vi "pmu_CFG-3 Dulplicate to CFG-2.vi"(8 "error in (no error)":errorcluster, 10 "CFG-3":T5={"PMU ID"=1, "global PMU ID"=1, "time base"=10000000, "nominal frequency"=enum."60 Hz", "reporting rate [fps]"=60, "station name"="", "data format"=15, "phasor channels"=[], "analog channels"=[], "digital channels"=[]} {"data format" format="%016b"; "phasor channels"."phasor unit" items=["Voltage [V]"=0, "Current [A]"=16777216]; "phasor channels"."data modification flag" format="%016b"; "digital channels"."digital unit" format="%08x"}, 11 "CFG-2":T1={"PMU ID"=1, "time base"=10000000, "nominal frequency"=enum."60 Hz", "reporting rate [fps]"=60, "station name"="", "data format"=15, "phasor channels"=[], "analog channels"=[], "digital channels"=[]} {"digital channels"."digital unit" format="%08x"; "analog channels"."analog unit" format="%08x"; "phasor channels"."phasor unit scaling" max=16777215 format="%06x"; "phasor channels"."phasor unit" items=["Voltage [V]"=0, "Current [A]"=16777216]; "data format" format="%016b"}) -> (0 "error out":errorcluster, 3 "CFG-2 output":T1={"PMU ID"=0, "time base"=10000000, "nominal frequency"=enum."60 Hz", "reporting rate [fps]"=60, "station name"="", "data format"=15, "phasor channels"=[], "analog channels"=[], "digital channels"=[]} {"digital channels"."digital unit" format="%08x"; "analog channels"."analog unit" format="%08x"; "phasor channels"."phasor unit scaling" max=16777215 format="%06x"; "phasor channels"."phasor unit" items=["Voltage [V]"=0, "Current [A]"=16777216]; "data format" format="%016b"})   [LabVIEW 2013, in "NI_EP_PMU.lvlib"]
uses:
  <vilib>/addons/Electrical Power/PMU/NI_EP_PMU.lvlib
  <vilib>/addons/Electrical Power/PMU/Common/Controls/pmu_CFG-3 Input.ctl
  <vilib>/addons/Electrical Power/PMU/Common/Controls/pmu_CFG-3 Phasor Channels.ctl
  <vilib>/addons/Electrical Power/PMU/Common/Controls/pmu_CFG-3 Analog Channels.ctl
  <vilib>/addons/Electrical Power/PMU/Common/Controls/pmu_Digital Channel.ctl
  <vilib>/addons/Electrical Power/PMU/Common/Controls/pmu_CFG Input.ctl
  <vilib>/addons/Electrical Power/PMU/Common/Controls/pmu_Phasor Channel.ctl
  <vilib>/addons/Electrical Power/PMU/Common/Controls/pmu_Analog Channel.ctl
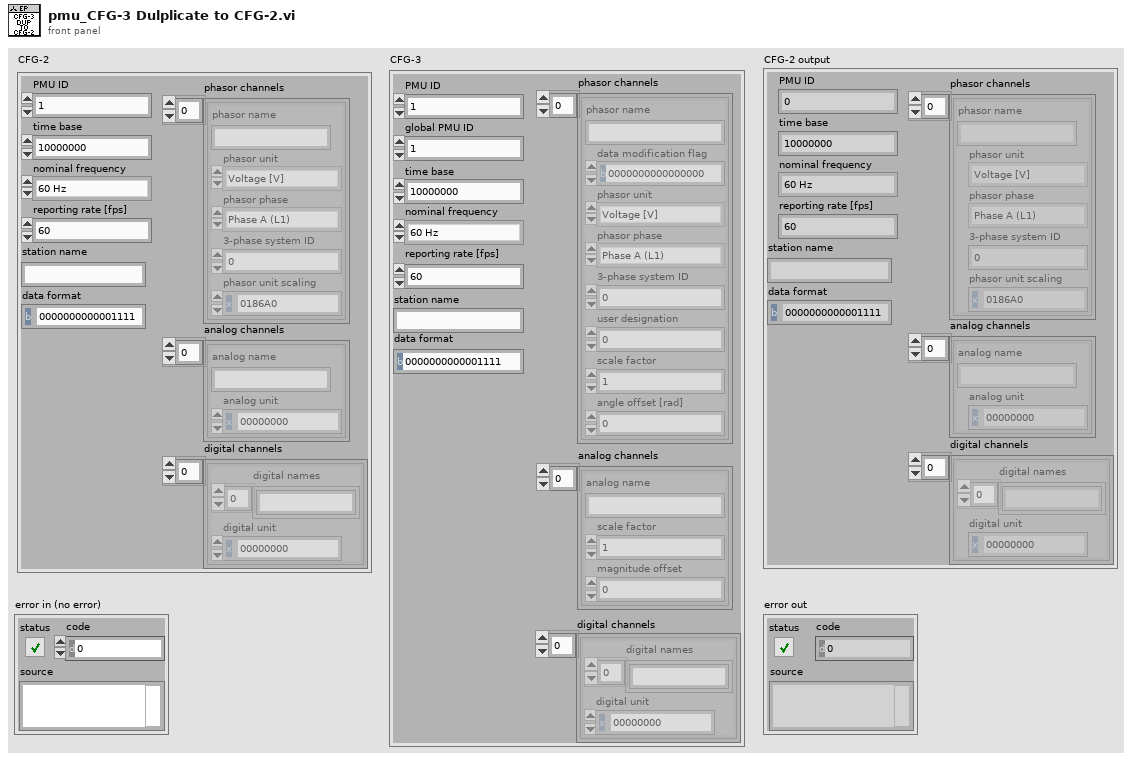
[diagram p1: front panel]
types:
  T1 = typedef "NI_EP_PMU.lvlib/pmu_CFG Input.ctl" = cluster{"PMU ID":u16, "time base":u32, "nominal frequency":enum16{"50 Hz", "60 Hz"}, "reporting rate [fps]":i16, "station name":string, "data format":u16, "phasor channels":T2[], "analog channels":T3[], "digital channels":T4[]}
  T2 = typedef "NI_EP_PMU.lvlib/pmu_Phasor Channel.ctl" = cluster{"phasor name":string, "phasor unit":u32, "phasor phase":enum16{"Phase A (L1)", "Phase B (L2)", "Phase C (L3)", "Phase N", "Positive sequence", "Negative sequence", "Zero sequence"}, "3-phase system ID":u8, "phasor unit scaling":u32}
  T3 = typedef "NI_EP_PMU.lvlib/pmu_Analog Channel.ctl" = cluster{"analog name":string, "analog unit":u32}
  T4 = typedef "NI_EP_PMU.lvlib/pmu_Digital Channel.ctl" = cluster{"digital names":string[], "digital unit":u32}
  T5 = typedef "NI_EP_PMU.lvlib/pmu_CFG-3 Input.ctl" = cluster{"PMU ID":u16, "global PMU ID":u64, "time base":u32, "nominal frequency":enum16{"50 Hz", "60 Hz"}, "reporting rate [fps]":i16, "station name":string, "data format":u16, "phasor channels":T6[], "analog channels":T7[], "digital channels":T4[]}
  T6 = typedef "NI_EP_PMU.lvlib/pmu_CFG-3 Phasor Channels.ctl" = cluster{"phasor name":string, "data modification flag":u16, "phasor unit":u32, "phasor phase":enum16{"Phase A (L1)", "Phase B (L2)", "Phase C (L3)", "Phase N", "Positive sequence", "Negative sequence", "Zero sequence"}, "3-phase system ID":u8, "user designation":u8, "scale factor":sgl, "angle offset [rad]":sgl}
  T7 = typedef "NI_EP_PMU.lvlib/pmu_CFG-3 Analog Channels.ctl" = cluster{"analog name":string, "scale factor":sgl, "magnitude offset":sgl}
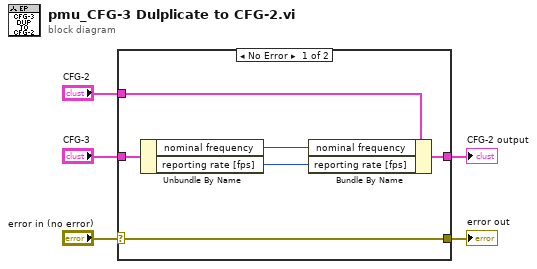
[diagram p0: block diagram]
diagram:
  n1 = case shown="No Error" "error in (no error)" {
    selector: "error in (no error)" -> [w6 w12]
    tunnel: "CFG-3" -> [w11 _]
    tunnel: "CFG-2" -> [w8 _]
    tunnel: [w7 _] -> w3
    tunnel: [w6 w12] -> w1
    frame No Error {
      n2 = Unbundle By Name(w11) -> ("nominal frequency"=w9:enum16{"50 Hz", "60 Hz"}, "reporting rate [fps]"=w10:i16)
      n3 = Bundle By Name(cluster=w8, "nominal frequency"=w9, "reporting rate [fps]"=w10) -> (w7:T1)
    }
    frame Error {
    }
  }
  "CFG-2 output" <- w3
  "error out" <- w1
